vi "Message updater.vi"(10 "Message Selector":T1) -> (2 "Message":string)   [LabVIEW 2019]
doc: "This VI is an FGV used to update display message."
uses:
  Controls/Message selector.ctl
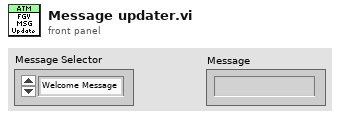
[diagram p1: front panel]
types:
  T1 = typedef "Message selector.ctl" = enum16{"Welcome Message", "Main Menu Message", "Account Verification Failed Message", "Session Terminate Message", "Deposit Message", "Deposit Complete Message", "Withdrawal Message", "Withdrawal Complete Message", "Withdrawal Failed Message", "Balance Inquiry Message"}
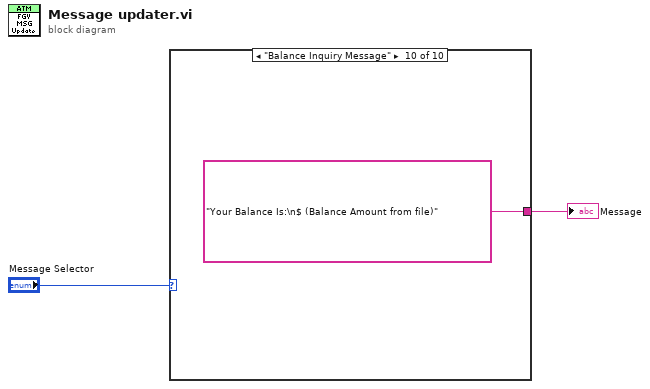
[diagram p0: block diagram]
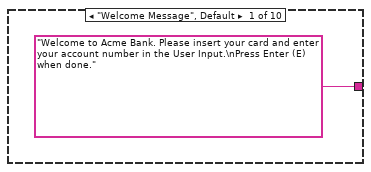
[diagram p2: hidden frame]
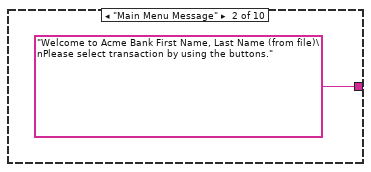
[diagram p3: hidden frame]
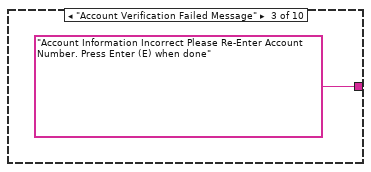
[diagram p4: hidden frame]
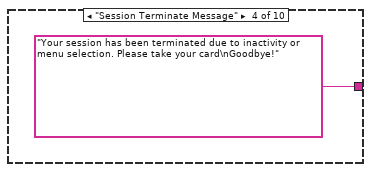
[diagram p5: hidden frame]
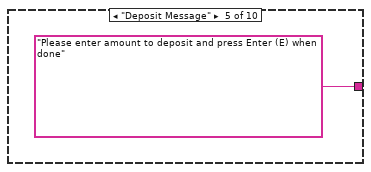
[diagram p6: hidden frame]
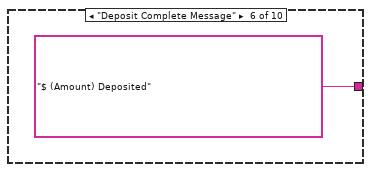
[diagram p7: hidden frame]
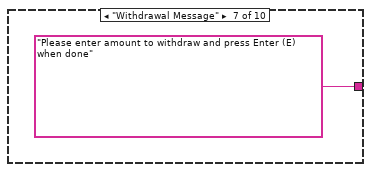
[diagram p8: hidden frame]
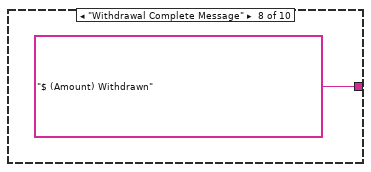
[diagram p9: hidden frame]
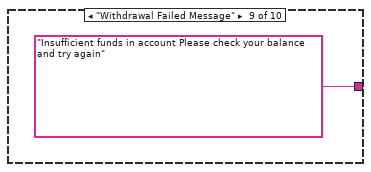
[diagram p10: hidden frame]
diagram:
  n1 = case shown="\"Balance Inquiry Message\"" "Message Selector" {
    tunnel: ["Welcome to Acme Bank. Please insert your card and enter your account number in the User Input.\nPress Enter (E) when done." "Welcome to Acme Bank First Name, Last Name (from file)\nPlease select transaction by using the buttons." "Account Information Incorrect Please Re-Enter Account Number. Press Enter (E) when done" "Your session has been terminated due to inactivity or menu selection. Please take your card\nGoodbye!" "Please enter amount to deposit and press Enter (E) when done" "$ (Amount) Deposited" "Please enter amount to withdraw and press Enter (E) when done" "$ (Amount) Withdrawn" "Insufficient funds in account Please check your balance and try again" "Your Balance Is:\n$ (Balance Amount from file)"] -> w1
    frame "Welcome Message", Default {
    }
    frame "Main Menu Message" {
    }
    frame "Account Verification Failed Message" {
    }
    frame "Session Terminate Message" {
    }
    frame "Deposit Message" {
    }
    frame "Deposit Complete Message" {
    }
    frame "Withdrawal Message" {
    }
    frame "Withdrawal Complete Message" {
    }
    frame "Withdrawal Failed Message" {
    }
    frame "Balance Inquiry Message" {
    }
  }
  "Message" <- w1
